vi "SetTimerResetCondition.vi"(2 "error in (no error)":errorcluster, 3 "Reset Timer Condition":u8(ring) items=["External Trigger In", "External Modulation In"], 4 "Timer Condition Status":bool, 5 "VISA resource name":refnum<visa-resource-name>) -> (0 "error out":errorcluster, 1 "VISA resource name out":refnum<visa-resource-name>)   [LabVIEW 2020, in "Active Technologies AWG3000.lvlib"]
uses:
  Active Technologies AWG3000.lvlib
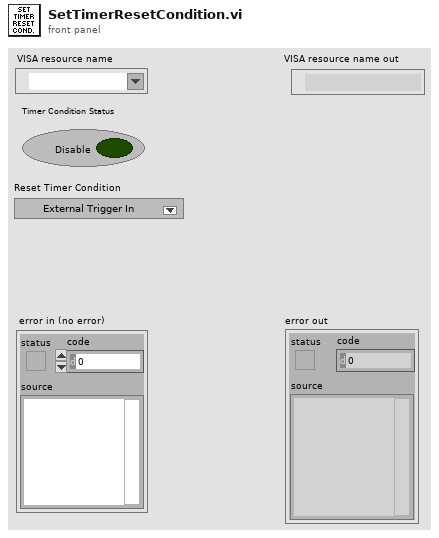
[diagram p1: front panel]
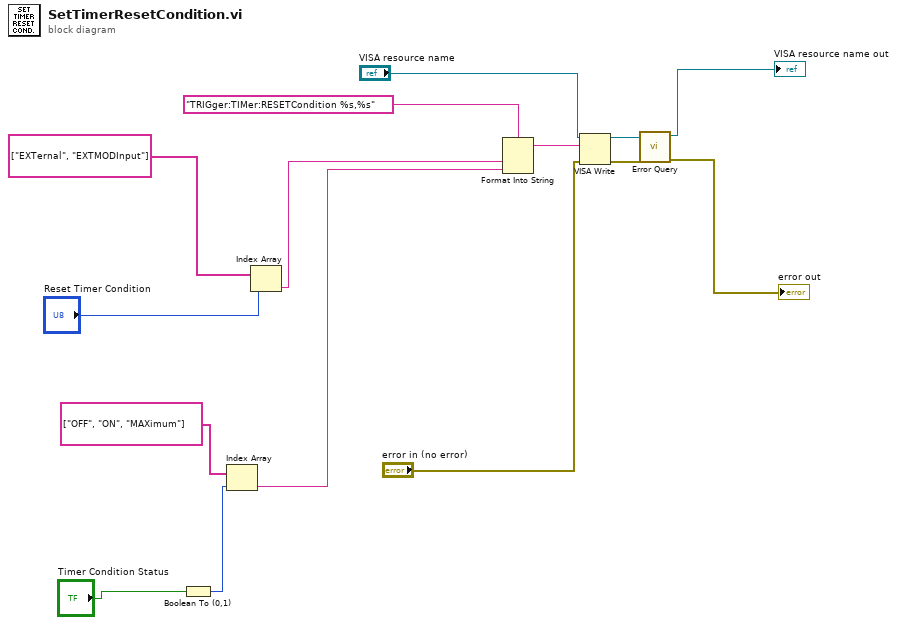
[diagram p0: block diagram]
diagram:
  n1 = Boolean To (0,1)(Boolean="Timer Condition Status") -> (0, 1=w4:i16)
  n2 = Index Array(array=string[] ["OFF", "ON", "MAXimum"], index=w4) -> (element=w1:string)
  n3 = Index Array(array=string[] ["EXTernal", "EXTMODInput"], index="Reset Timer Condition") -> (element=w5:string)
  n4 = Format Into String(format string="TRIGger:TIMer:RESETCondition %s,%s" ("write buffer"), w5, w1) -> (resulting string=w12:string)  [unwired: 2 in, 1 out]
  n5 = VISA Write(VISA resource name="VISA resource name", write buffer=w12, error in (no error)="error in (no error)") -> (VISA resource name out=w11:refnum<visa-resource-name>, error out=w10:errorcluster)  [unwired: 1 out]
  n6 = call "Error Query.vi"("error in (no error)"=w10, "VISA resource name"=w11) -> ("error out"=→"error out":errorcluster, "VISA resource name out"=→"VISA resource name out":refnum<visa-resource-name>)  [unwired: 6 in, 2 out]
